vi "DSF.Engine.Transceiver.Command.Receive.vi"(8 "error in (no error)":errorcluster, 9 "timeout in ms (0)":i32 format="%d ms", 11 "Transceiver Thread in":refnum<class "DSF.Engine.Transceiver Thread.lvclass">) -> (0 "error out":errorcluster, 1 "timed out?":bool, 2 "command":T1={"Command"=enum."Rx", "Command Parameters"={"arg1"=0, "arg2"=0}}, 3 "Transceiver Thread out":refnum<class "DSF.Engine.Transceiver Thread.lvclass">)   [LabVIEW 2017, in "DSF.Engine.lvlib" / "DSF.Engine.Transceiver Thread.lvclass"]
uses:
  DSF.Engine.Transceiver Thread.lvclass
  Interface/DSF.Engine.Interface.Transceiver.Command Data.ctl
  Interface/DSF.Engine.Interface.Transceiver.Command.ctl
  Interface/DSF.Engine.Interface.Transceiver.Command Parameters.ctl
  DSF.Engine.Transceiver Thread.lvclass/DSF.Engine.Transceiver Thread.ctl
  Interface/DSF.Engine.Interface.lvclass/DSF.Engine.Interface.ctl
  Debug/DSF.Engine.Debug Flags.FIFO.lvclass/DSF.Engine.Debug Flags.FIFO.ctl
  Interface/DSF.Engine.Interface.Transceiver.Read.Command.vi
  Interface/DSF.Engine.Interface.Read.Command.vi
  Interface/DSF.Engine.Interface.Get Command FIFO.vi
  Interface/DSF.Engine.Interface.Get Debug Flags.vi
  Interface/DSF.Engine.Interface.RT FIFO.Read.16B.vi
  Debug/DSF.Engine.Debug Flags.FIFO.Get Infinite Timeouts.vi
  Interface/DSF.Engine.Interface.Transceiver.lvclass
  C:/Git/DSF/dsf core/Source/Engine/Classes/Interface/DSF.Engine.Interface.lvclass
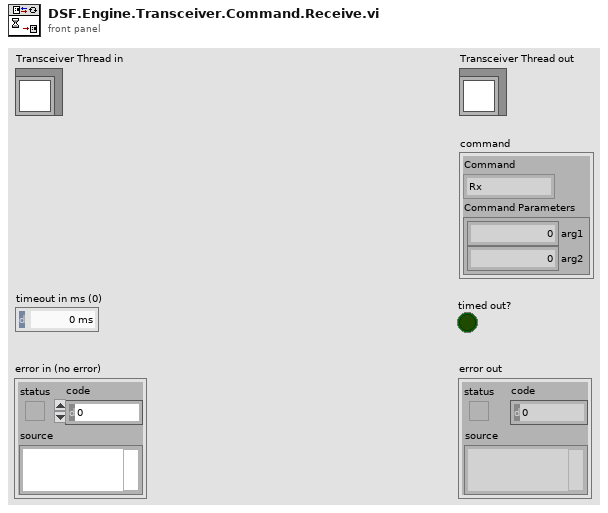
[diagram p1: front panel]
types:
  T1 = typedef "DSF.Engine.lvlib/DSF.Engine.Interface.Transceiver.lvclass/DSF.Engine.Interface.Transceiver.Command Data.ctl" = cluster{"Command":T2, "Command Parameters":T3}
  T2 = typedef "DSF.Engine.lvlib/DSF.Engine.Interface.Transceiver.lvclass/DSF.Engine.Interface.Transceiver.Command.ctl" = enum8{"Set Base Pointer", "Rx", "Tx", "Shutdown"}
  T3 = typedef "DSF.Engine.lvlib/DSF.Engine.Interface.Transceiver.lvclass/DSF.Engine.Interface.Transceiver.Command Parameters.ctl" = cluster{"arg1":u64, "arg2":u64}
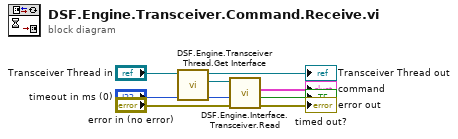
[diagram p0: block diagram]
diagram:
  n1 = call "DSF.Engine.Transceiver Thread.Get Interface.vi"("Transceiver Thread in"="Transceiver Thread in") -> ("Interface"=w7:refnum<class "DSF.Engine.Interface.Transceiver.lvclass">, "Transceiver Thread out"=→"Transceiver Thread out":refnum<class "DSF.Engine.Transceiver Thread.lvclass">)  [unwired: 9 in]
  n2 = call-poly "DSF.Engine.Interface.Transceiver.Read.vi"("error in (no error)"="error in (no error)", "timeout in ms (0)"="timeout in ms (0)", "Transceiver Interface in"=w7) -> ("error out"=→"error out":errorcluster, "empty?"=→"timed out?":bool, "command"=→"command":T1)  [unwired: 4 in, 2 out]
